vi "GetTachometerChannelProperties.vi"(11 "Channel":T1) -> (3 "Tachometer Properties":T4[](array[typedef]))   [LabVIEW 2017, in "Tdms.lvlib"]
uses:
  <vilib>/addons/InsightCM/Utilities/Tdms/Tdms.lvlib
  <vilib>/addons/InsightCM/Utilities/Tdms/controls/Property.ctl
  <vilib>/addons/InsightCM/MessageBus/Base/controls/R2_Channel.ctl
  <vilib>/addons/InsightCM/MessageBus/Base/controls/KeyValuePair.ctl
  <vilib>/addons/InsightCM/MessageBus/Base/controls/Metric.ctl
  <vilib>/addons/InsightCM/Utilities/PropertyHelpers/PropertyHelpers.lvlib
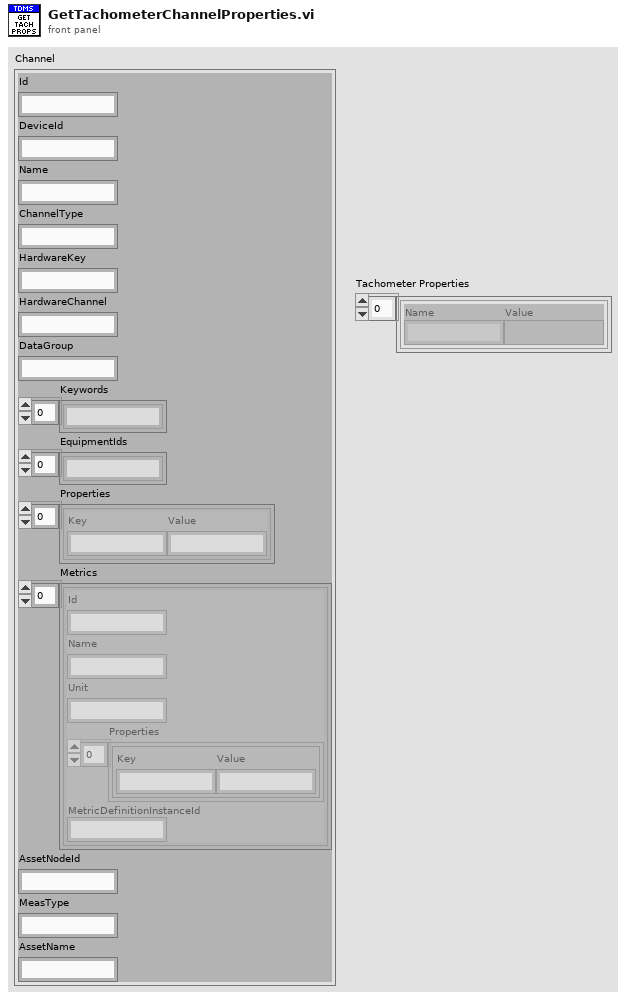
[diagram p1: front panel]
types:
  T1 = typedef "R2_Channel.ctl" = cluster{"Id":string, "DeviceId":string, "Name":string, "ChannelType":string, "HardwareKey":string, "HardwareChannel":string, "DataGroup":string, "Keywords":string[], "EquipmentIds":string[], "Properties":T2[], "Metrics":T3[], "AssetNodeId":string, "MeasType":string, "AssetName":string}
  T2 = typedef "KeyValuePair.ctl" = cluster{"Key":string, "Value":string}
  T3 = typedef "Metric.ctl" = cluster{"Id":string, "Name":string, "Unit":string, "Properties":T2[], "MetricDefinitionInstanceId":string}
  T4 = typedef "Tdms.lvlib/Property.ctl" = cluster{"Name":string, "Value":variant}
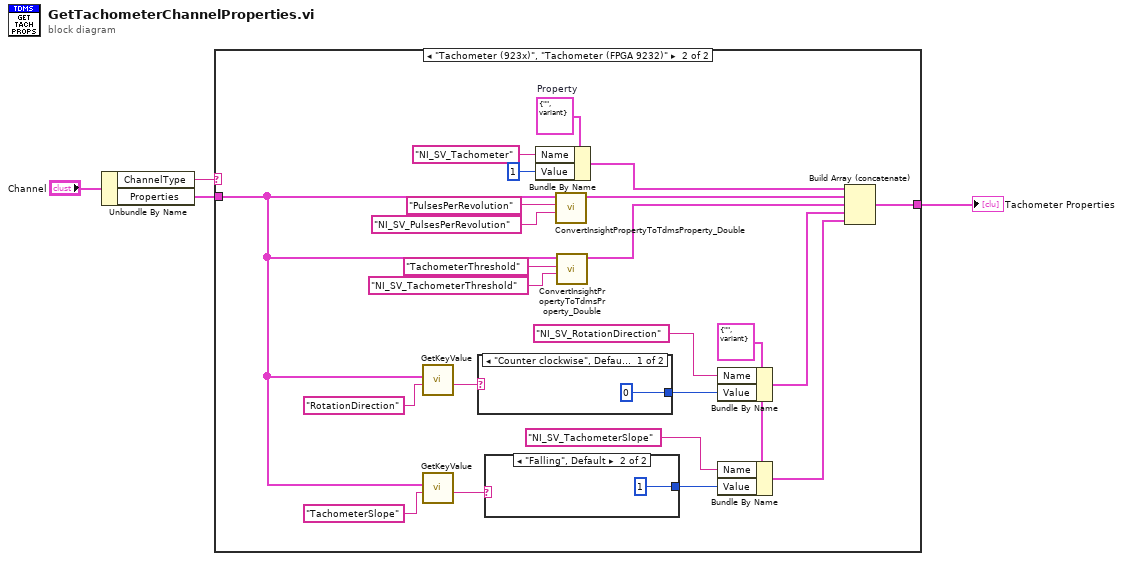
[diagram p0: block diagram]
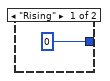
[diagram p3: hidden frame]
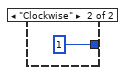
[diagram p4: hidden frame]
diagram:
  n1 = Unbundle By Name("Channel") -> ("ChannelType"=w2:string, "Properties"=w1:T2[])
  n2 = case shown="\"Tachometer (923x)\", \"Tachometer (FPGA 9232)\"" w2 {
    tunnel: [_ w14] -> w4
    tunnel: w1 -> [_ w7]
    frame Default {
    }
    frame "Tachometer (923x)", "Tachometer (FPGA 9232)" {
      w19 = T4 {"Name"="", "Value"=variant} ("Property")
      w22 = T4 {"Name"="", "Value"=variant}  # Property
      n3 = call <vilib>:"GetKeyValue.vi"("key"="RotationDirection" ("Name"), "key value pairs"=w7) -> ("value"=w10:string)  [unwired: 7 in, 2 out]
      n4 = call <vilib>:"GetKeyValue.vi"("key"="TachometerSlope" ("Name"), "key value pairs"=w7) -> ("value"=w9:string)  [unwired: 7 in, 2 out]
      n5 = case shown="\"Counter clockwise\", Default" w10 {
        tunnel: [0 ("number") 1 ("number")] -> w20
        frame "Counter clockwise", Default {
        }
        frame "Clockwise" {
        }
      }
      n6 = case shown="\"Falling\", Default" w9 {
        tunnel: [0 ("number") 1 ("number")] -> w21
        frame "Rising" {
        }
        frame "Falling", Default {
        }
      }
      n7 = Bundle By Name(cluster=w22, "Name"="NI_SV_Tachometer", "Value"=1 ("number")) -> (w27:T4)
      n8 = call <vilib>:"ConvertInsightPropertyToTdmsProperty_Double.vi"("Tdms Property Name"="NI_SV_PulsesPerRevolution" ("Name"), "Insight Property Name"="PulsesPerRevolution" ("Name"), "Insight Properties"=w7) -> ("Tdms Properties"=w8:T4[])  [unwired: 8 in]
      n9 = call <vilib>:"ConvertInsightPropertyToTdmsProperty_Double.vi"("Tdms Property Name"="NI_SV_TachometerThreshold" ("Name"), "Insight Property Name"="TachometerThreshold" ("Name"), "Insight Properties"=w7) -> ("Tdms Properties"=w15:T4[])  [unwired: 8 in]
      n10 = Bundle By Name(cluster=w19, "Name"="NI_SV_RotationDirection", "Value"=w20) -> (w16:T4)
      n11 = Bundle By Name(cluster=w19, "Name"="NI_SV_TachometerSlope", "Value"=w21) -> (w23:T4)
      n12 = Build Array (concatenate)(w27, w8, w15, w16, w23) -> (w14:T4[])
    }
  }
  "Tachometer Properties" <- w4
